vi "Streamed to Waveform Converter.vi"() -> ()   [LabVIEW 2013]
doc: "Use this template to build a user interface event handler design pattern. Use this pattern for dialog boxes and other user interfaces. You also can create and execute user-defined events that the VI can handle the same way as user interface events."
uses:
  <vilib>/Waveform/WDTFileIO.llb/ Write Waveforms to File (1D).vi
panel:
  out "Record Index":i32
  out "Streamed Data":dbl[][](graph)
  out "Waveform Data":waveform(dbl)[](graph)
  out "Output Path":path
  out "Record Count":u32
  in  "Sampling Rate":u32=500000
  in  "Record Channel Size":bool
  in  "Path":path
  in  "Convert":bool
  in  "stop":bool
  # "51200"
  # "51200 x 3"
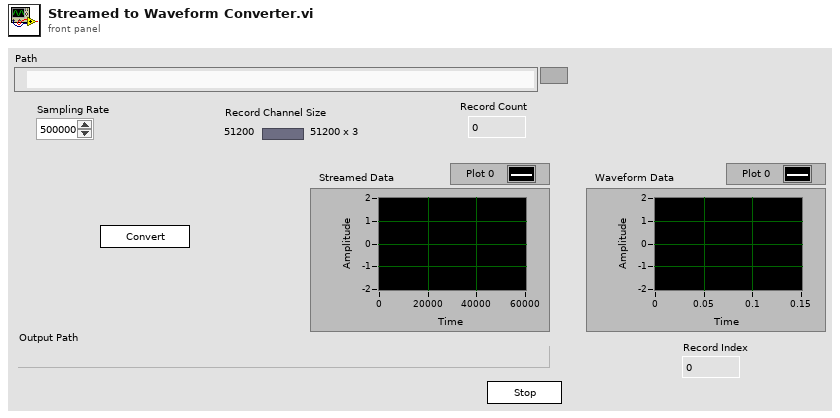
[diagram p1: front panel]
types:
  T1 = enum16{"big-endian, network order", "native, host order", "little-endian"}
  T2 = enum16{"open", "replace", "create", "open or create", "replace or create", "replace or create with confirmation"}
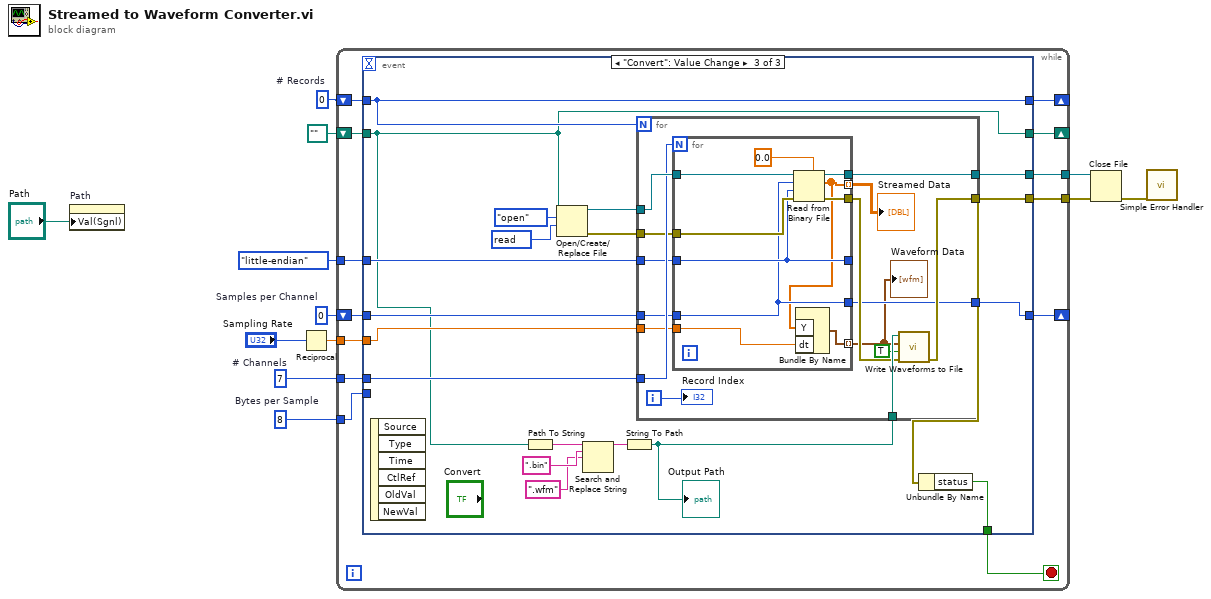
[diagram p0: block diagram]
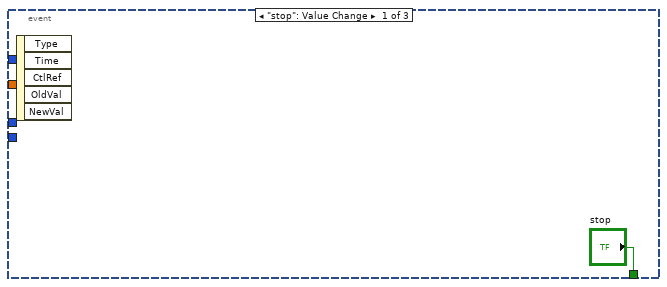
[diagram p2: hidden frame]
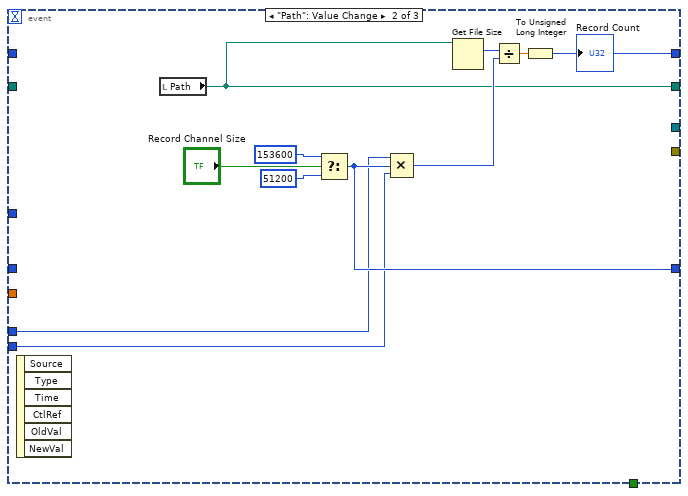
[diagram p3: hidden frame]
diagram:
  w8 = u32 8  # Bytes per Sample
  w9 = u32 7  # # Channels
  w10 = u32 0  # Samples per Channel
  w12 = u32 0  # # Records
  n1 = property on="Path" class="Path"("Val(Sgnl)"="Path") -> ()  [unwired: 2 in, 2 out]
  n2 = Reciprocal(x="Sampling Rate") -> (1/x=w6:dbl)
  n3 = while {
    shift-right: [w24] -> _
    shift-left: w12 -> [w23]
    shift-right: [w22] -> _
    shift-left: path "" ("Path") -> [w21]
    shift-right: [w20] -> _
    shift-left: w10 -> [w19]
    tunnel: w9 -> [w18]
    tunnel: w8 -> [w17]
    tunnel: w6 -> [w16]
    tunnel: T1."little-endian" ("byte order (0:big-endian, network order)") -> [w15]
    tunnel: [w14] -> w4
    tunnel: [w13] -> w3
    stop <- w25 stop-if-true
    n4 = event shown="[2] \"Convert\": Value Change" {
      selector: _ -> [_ _ _]
      dyn-events: _ -> [_ _ _]
      timeout: _ -> [_ _ _]
      tunnel: ["stop" _ w40] -> w25
      tunnel: [_ w36 w45] -> w24
      tunnel: w23 -> [_ _ w45]
      tunnel: [_ w29 w44] -> w22
      tunnel: w21 -> [_ _ w44]
      tunnel: [_ w32 w43] -> w20
      tunnel: w19 -> [_ _ w49]
      tunnel: w18 -> [_ w31 w50]
      tunnel: w17 -> [_ w30 _]
      tunnel: w16 -> [_ _ w48]
      tunnel: w15 -> [_ _ w47]
      tunnel: [_ _ w46] -> w14
      tunnel: [_ _ w41] -> w13
      event "stop": Value Change {
        n5 = event-data() -> ()  [unwired: 1 in, 5 out]
      }
      event "Path": Value Change {
        n6 = event-data() -> ()  [unwired: 1 in, 6 out]
        n7 = local read "Path"() -> (w29:path)
        n8 = Select(t=u32 153600, s="Record Channel Size", f=u32 51200) -> (s? t:f=w32:u32)
        n9 = Compound Arithmetic op=MULTIPLY(w31, w32, w30) -> (w33:u32)
        n10 = Get File Size(file=w29) -> (size (in bytes)=w34:i64)  [unwired: 1 in, 2 out]
        n11 = Divide(x=w34, y=w33) -> (x/y=w35:dbl)
        n12 = To Unsigned Long Integer(number=w35) -> (unsigned 32bit integer=w36:u32)
        "Record Count" <- w36
      }
      event "Convert": Value Change {
        w56 = u32 2147483648 items=["read"=2147483648, "write"=1073741824, "read & write"=3221225472, "execute"=536870912, "all"=268435456] ("desired access (read & write)")
        n13 = event-data() -> ()  [unwired: 1 in, 6 out]
        n14 = Path To String(path=w44) -> (string=w55:string)
        n15 = Open/Create/Replace File(file path (use dialog)=w44, operation (0:open)=T2."open", access (0:read/write)=w56) -> (refnum out=w51:refnum<file>, error out=w39:errorcluster)  [unwired: 3 in, 1 out]
        n16 = Search and Replace String(input string=w55, search string=".bin", replace string=".wfm" ("replace string (\"\")")) -> (result string=w52:string)  [unwired: 5 in, 3 out]
        n17 = String To Path(string=w52) -> (path=w38:path)
        "Output Path" <- w38
        n18 = for {
          N: w45 -> [_]
          tunnel: w51 -> [w71]
          tunnel: w50 -> [w70]
          tunnel: w49 -> [w69]
          tunnel: w39 -> [w68]
          tunnel: w48 -> [w67]
          tunnel: w47 -> [w66]
          tunnel: w38 -> [w65]
          tunnel: [w63] -> w46
          tunnel: [w62] -> w41
          tunnel: [w61] -> w43
          i -> [w57]
          n19 = for {
            N: w70 -> [_]
            tunnel: [w81] -> w60 mode=indexing
            tunnel: w71 -> [w79]
            tunnel: w69 -> [w73]
            tunnel: w68 -> [w78]
            tunnel: w67 -> [w77]
            tunnel: w66 -> [w75]
            tunnel: [w76] -> w64
            tunnel: [w75] -> _
            tunnel: [w74] -> w63
            tunnel: [w73] -> w61
            tunnel: [w72] -> w59 mode=indexing
            n20 = Read from Binary File(5:0.0, 8:w78, 9:w75, 10:w73, 11:w79) -> (0:w76:errorcluster, 2:w72:dbl[], 3:w74:refnum<file>)  [unwired: 1 in, 1 out]
            n21 = Bundle By Name("Y"=w72, "dt"=w77) -> (w81:waveform(dbl))  [unwired: 1 in]
          }
          "Waveform Data" <- w60
          "Streamed Data" <- w59
          n22 = call-poly <vilib>:"Write Waveforms to File.vi"("error in (no error)"=w64, "append to file? (new file:F)"=TRUE, "waveform array"=w60, "file path (dialog if empty)"=w65) -> ("error out"=w62:errorcluster)  [unwired: 6 in, 1 out]
          "Record Index" <- w57
        }
        n23 = Unbundle By Name(w41) -> ("status"=w40:bool)
      }
    }
  }
  n24 = Close File(refnum=w4, error in=w3) -> (error out=w1:errorcluster)  [unwired: 1 out]
  n25 = call <vilib>:"Simple Error Handler.vi"("error in (no error)"=w1) -> ()  [unwired: 4 in, 5 out]
